vi "rad_FTP Delete File Wrapper.vi"(5 "password":string, 6 "timeout ms (500)":i32=500, 7 "user (admin)":string="admin", 8 "error in (no error)":errorcluster, 10 "remote path":string, 11 "Target settings":T1={"Hostname"="", "Serial number"="", "Product name"="", "Product code"=0, "System status"="", "Credential type"=enum."None/Unlocked", "User added?"=FALSE, "Primary NIC"={"MAC address"="", "IP Address Request Mode"=2, "IP address"="", "Subnet mask"="", "Gateway"="", "DNS server"=""}} {"Primary NIC"."IP Address Request Mode" items=["Static"=1, "DHCP/Link-Local"=2, "Link-Local Only"=4, "DHCP Only"=8]}) -> (0 "error out":errorcluster)   [LabVIEW 2020]
uses:
  support/SubVIs/Target Information.ctl
  Targets/TypeDefs/rad_Target Network Settings.ctl
  <vilib>/nisyscfg/Close (System).vi
  <vilib>/nisyscfg/nisyscfg.lvlib
  <vilib>/FTP/NI_FTP.lvlib
panel:
  out "reply string 2":string
  out "reply string":string
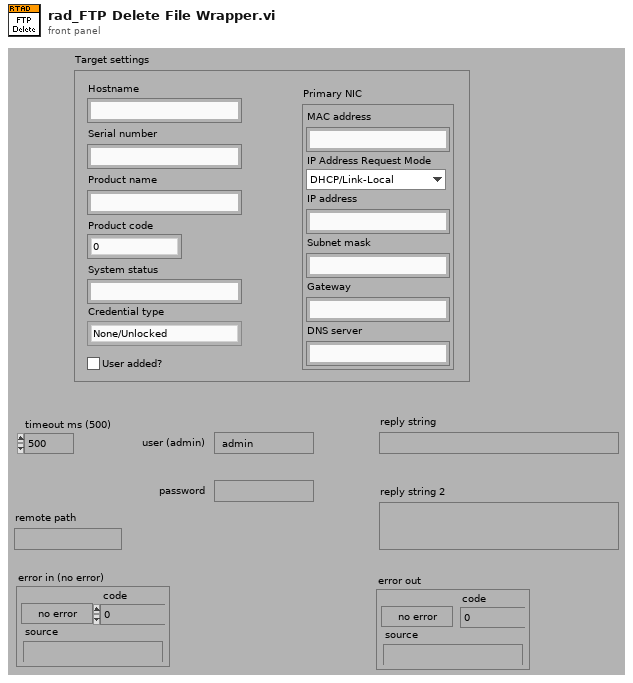
[diagram p1: front panel]
types:
  T1 = typedef "Target Information.ctl" = cluster{"Hostname":string, "Serial number":string, "Product name":string, "Product code":i32, "System status":string, "Credential type":enum16{"None/Unlocked", "FTP Password", "NIAuth Credentials"}, "User added?":bool, "Primary NIC":T2}
  T2 = typedef "rad_Target Network Settings.ctl" = cluster{"MAC address":string, "IP Address Request Mode":i32, "IP address":string, "Subnet mask":string, "Gateway":string, "DNS server":string}
  T3 = typedef "NI_FTP.lvlib/FTP Session.ctl" = refnum<k5>
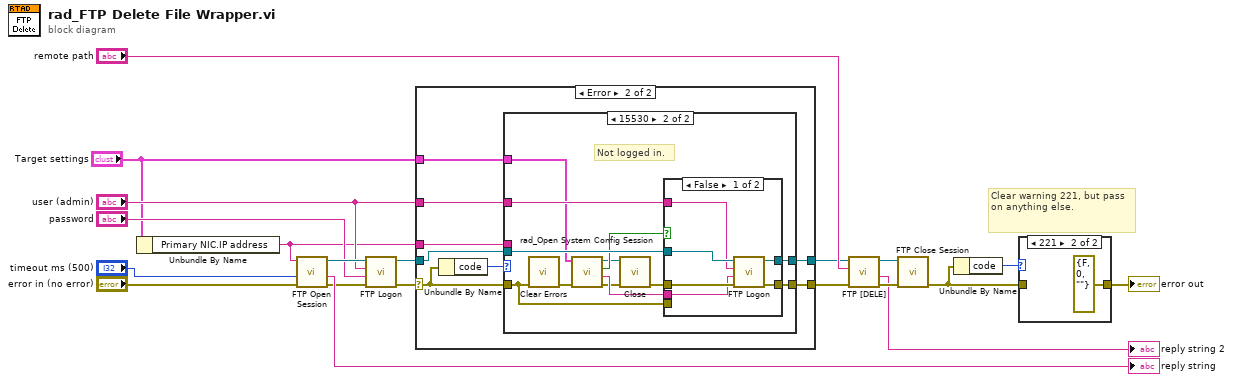
[diagram p0: block diagram]
diagram:
  # "Clear warning 221, but pass on anything else."
  n1 = Unbundle By Name("Target settings") -> ("Primary NIC.IP address"=w2:string)
  n2 = call <vilib>:"FTP Open Session.vi"("error in (no error)"="error in (no error)", "timeout ms (60000)"="timeout ms (500)", "address"=w2) -> ("error out"=w4:errorcluster, "reply string"=→"reply string":string, "ftp session"=w14:T3)  [unwired: 5 in, 1 out]
  n3 = call <vilib>:"FTP Logon.vi"("error in (no error)"=w4, "password"="password", "user"="user (admin)", "ftp session"=w14) -> ("error out"=w9:errorcluster, "ftp session out"=w8:T3)  [unwired: 4 in, 2 out]
  n4 = case shown="Error" w9 {
    selector: w9 -> [w22 w26]
    tunnel: [w22 w28] -> w6
    tunnel: w8 -> [w21 w29]
    tunnel: [w21 w27] -> w7
    tunnel: w2 -> [_ w30]
    tunnel: "user (admin)" -> [_ w24]
    tunnel: "Target settings" -> [_ w23]
    frame No Error {
    }
    frame Error {
      n5 = Unbundle By Name(w26) -> ("code"=w25:i32)
      n6 = case shown="15530" w25 {
        tunnel: w30 -> [_ _]
        tunnel: w26 -> [w32 w41]
        tunnel: w29 -> [w31 w43]
        tunnel: [w32 w42] -> w28
        tunnel: [w31 w40] -> w27
        tunnel: w24 -> [_ w34]
        tunnel: w23 -> [_ w33]
        frame Default {
        }
        frame 15530 {
          # "Not logged in."
          n7 = call <vilib>:"Clear Errors.vi"("error in (no error)"=w41) -> ("error out"=w39:errorcluster)  [unwired: 5 in, 1 out]
          n8 = call "rad_Open System Config Session.vi"("error in (no error)"=w39, "Target settings"=w33) -> ("error out"=w35:errorcluster, "Password out"=w36:string, "Cancelled"=w38:bool, "Session out"=w37:refnum<k21>)  [unwired: 6 in]
          n9 = call-poly <vilib>:"Close.vi"("error in (no error)"=w35, "Session in"=w37) -> ("error out"=w44:errorcluster)  [unwired: 9 in]
          n10 = case shown="False" w38 {
            tunnel: w44 -> [w50 _]
            tunnel: w43 -> [w49 w51]
            tunnel: [w48 w52] -> w42
            tunnel: w41 -> [_ w52]
            tunnel: [w47 w51] -> w40
            tunnel: w36 -> [w46 _]
            tunnel: w34 -> [w45 _]
            frame False {
              n11 = call <vilib>:"FTP Logon.vi"("error in (no error)"=w50, "password"=w46, "user"=w45, "ftp session"=w49) -> ("error out"=w48:errorcluster, "ftp session out"=w47:T3)  [unwired: 4 in, 2 out]
            }
            frame True {
            }
          }
        }
      }
    }
  }
  n12 = call <vilib>:"FTP [DELE].vi"("error in (no error)"=w6, "file path"="remote path", "ftp session"=w7) -> ("error out"=w18:errorcluster, "reply string"=→"reply string 2":string, "ftp session out"=w19:T3)  [unwired: 5 in, 1 out]
  n13 = call <vilib>:"FTP Close Session.vi"("error in (no error)"=w18, "ftp session"=w19) -> ("error out"=w11:errorcluster)  [unwired: 6 in, 3 out]
  n14 = Unbundle By Name(w11) -> ("code"=w12:i32)
  n15 = case shown="221" w12 {
    tunnel: [w53 errorcluster {"status"=FALSE, "code"=0, "source"=""} ("error IO")] -> w10
    tunnel: w11 -> [w53 _]
    frame Default {
    }
    frame 221 {
    }
  }
  "error out" <- w10
